vi "Case_structures.vi"() -> ()   [LabVIEW 2017]
panel:
  out "Random Value":dbl
  in  "Generate Random value?":bool
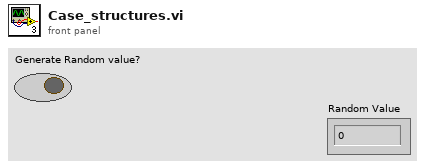
[diagram p1: front panel]
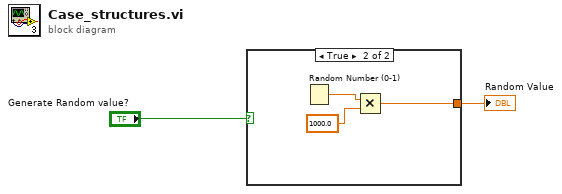
[diagram p0: block diagram]
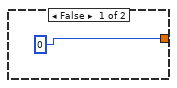
[diagram p2: hidden frame]
diagram:
  n1 = case shown="True" "Generate Random value?" {
    tunnel: [0 w4] -> w2
    frame False {
    }
    frame True {
      n2 = Random Number (0-1)() -> (number: 0 to 1=w6:dbl)
      n3 = Multiply(x=w6, y=1000.0) -> (x*y=w4:dbl)
    }
  }
  "Random Value" <- w2
